vi "Drive Slew Filter.vi"(8 "Slew Rate Filter Active?":bool, 9 "Precision Button":bool, 10 "Y Axis":dbl, 11 "X Axis":dbl) -> (2 "Y Axis Output":dbl, 3 "X Axis Output":dbl)   [LabVIEW 2014]
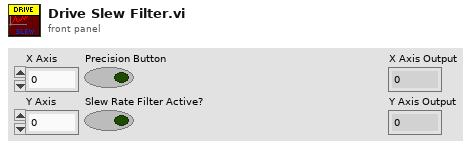
[diagram p1: front panel]
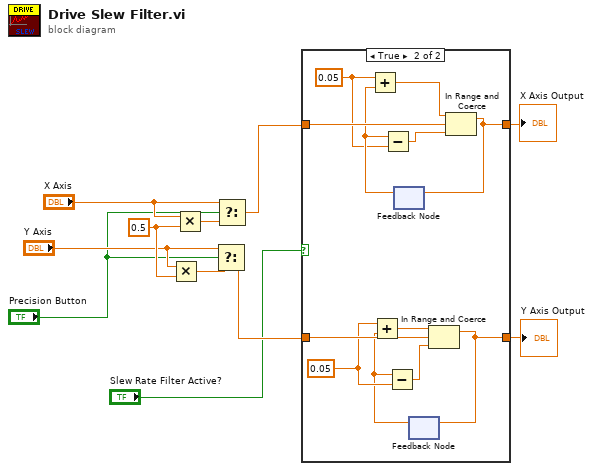
[diagram p0: block diagram]
diagram:
  w9 = 0.5 ("y")
  n1 = Multiply(x="Y Axis", y=w9) -> (x*y=w10:dbl)
  n2 = Multiply(x="X Axis", y=w9) -> (x*y=w11:dbl)
  n3 = Select(t="Y Axis", s="Precision Button", f=w10) -> (s? t:f=w5:dbl)
  n4 = Select(t="X Axis", s="Precision Button", f=w11) -> (s? t:f=w4:dbl)
  n5 = case shown="True" "Slew Rate Filter Active?" {
    tunnel: w5 -> [w12 w25]
    tunnel: w4 -> [w13 w24]
    tunnel: [w13 w15] -> w2
    tunnel: [w12 w14] -> w1
    frame False {
    }
    frame True {
      w20 = 0.05 ("x")
      w18 = 0.05 ("x")
      n6 = feedback #1() -> (w21:dbl)  [unwired: 1 in]
      n7 = Add(x=w20, y=w21) -> (x+y=w23:dbl)
      n8 = Subtract(x=w21, y=w20) -> (x-y=w22:dbl)
      n9 = feedback #2() -> (w17:dbl)  [unwired: 1 in]
      n10 = Add(x=w18, y=w17) -> (x+y=w16:dbl)
      n11 = Subtract(x=w17, y=w18) -> (x-y=w19:dbl)
      n12 = In Range and Coerce(upper limit=w16, x=w25, lower limit=w19) -> (coerced(x)=w14:dbl)  [unwired: 1 out]
      n13 = feedback-in #2(w14) -> ()
      n14 = In Range and Coerce(upper limit=w23, x=w24, lower limit=w22) -> (coerced(x)=w15:dbl)  [unwired: 1 out]
      n15 = feedback-in #1(w15) -> ()
    }
  }
  "X Axis Output" <- w2
  "Y Axis Output" <- w1
